vi "Facade.vi"(0 "Data In":T5, 2 "Display State In":T2={"WebView2 Ref"=refnum, "event callback refnum"=refnum, "Events"={"Navigation Complete Event"=refnum, "Source Changed Event"=refnum, "Document Title Changed Event"=refnum, "Status Bar Text Changed"=refnum, "Web Message Received"=refnum, "Window Close Requested"=refnum}, "Paths"={"Webview2 Native"=path "C:/Users/kleins/Desktop/webview2/microsoft.web.webview2.1.0.1370.28/build/native", "Edge Application"=path "", "User Data"=path ""}}, 3 "Container State":T4) -> (6 "Data Out":T5, 7 "Display State Out":T2={"WebView2 Ref"=refnum, "event callback refnum"=refnum, "Events"={"Navigation Complete Event"=refnum, "Source Changed Event"=refnum, "Document Title Changed Event"=refnum, "Status Bar Text Changed"=refnum, "Web Message Received"=refnum, "Window Close Requested"=refnum}, "Paths"={"Webview2 Native"=path "C:/Users/kleins/Desktop/webview2/microsoft.web.webview2.1.0.1370.28/build/native", "Edge Application"=path "", "User Data"=path ""}}, 8 "Action":T1)   [LabVIEW 2020, in "WebView2 Control.xctl"]
uses:
  WebView2 Control.xctl
  Data.ctl
  <vilib>/_xctls/Container State.ctl
  State.ctl
  C:/Users/kleins/Desktop/webview2/microsoft.web.webview2.1.0.1370.28/lib/net45/Microsoft.Web.WebView2.WinForms.dll
  microsoft.web.webview2.1.0.1370.28/lib/net45/Microsoft.Web.WebView2.WinForms.dll
  Paths.ctl
  <vilib>/_xctls/Action.ctl
  C:/Users/kleins/Desktop/webview2/microsoft.web.webview2.1.0.1370.28/lib/net45/Microsoft.Web.WebView2.Core.dll
  microsoft.web.webview2.1.0.1370.28/lib/net45/Microsoft.Web.WebView2.Core.dll
  <vilib>/_xctls/XControlSupport.lvlib
panel:
  in  "WebView2":refnum<k24>(container)
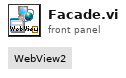
[diagram p1: front panel]
types:
  T1 = typedef "XControlSupport.lvlib/Action.ctl" = cluster{"Data Changed?":bool, "State Changed?":bool, "Action Name":string}
  T2 = typedef "WebView2 Control.xctl/State.ctl" = cluster{"WebView2 Ref":refnum<data-value>, "event callback refnum":refnum<k27>, "Events":cluster{"Navigation Complete Event":refnum<user-event>, "Source Changed Event":refnum<user-event>, "Document Title Changed Event":refnum<user-event>, "Status Bar Text Changed":refnum<user-event>, "Web Message Received":refnum<user-event>, "Window Close Requested":refnum<user-event>}, "Paths":T3}
  T3 = typedef "WebView2 Control.xctl/Paths.ctl" = cluster{"Webview2 Native":path, "Edge Application":path, "User Data":path}
  T4 = typedef "XControlSupport.lvlib/Container State.ctl" = cluster{"Indicator?":bool, "Run Mode?":bool, " Refnum":refnum<vi>}
  T5 = typedef "WebView2 Control.xctl/Data.ctl" = string
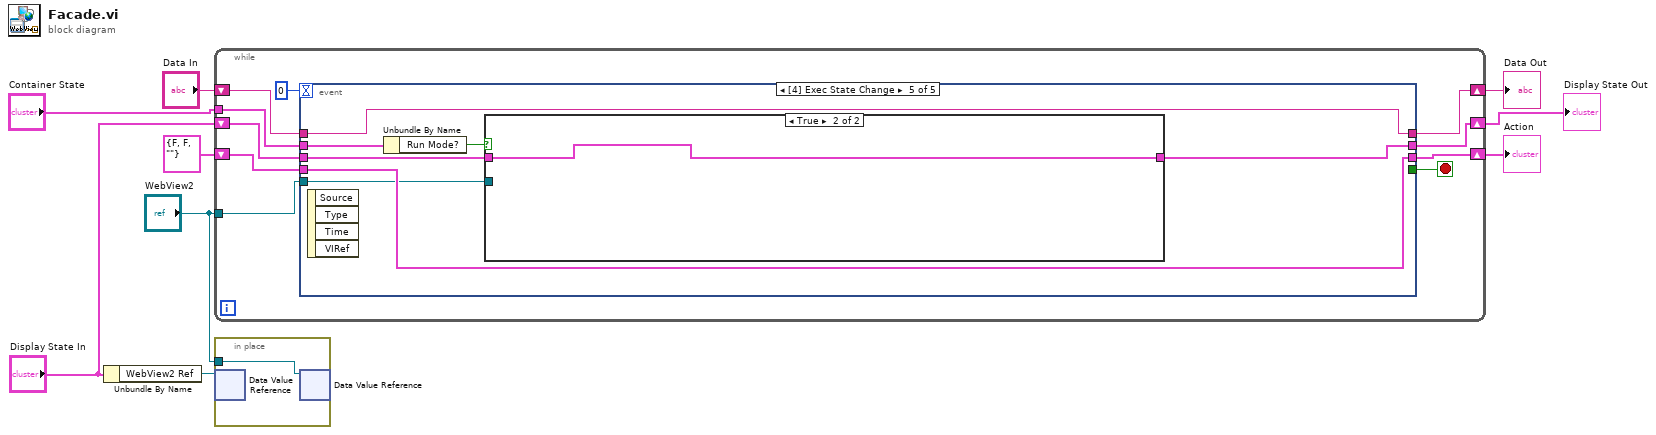
[diagram p0: block diagram]
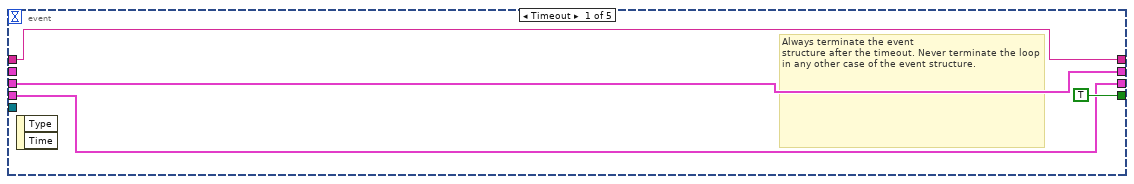
[diagram p2: hidden frame]
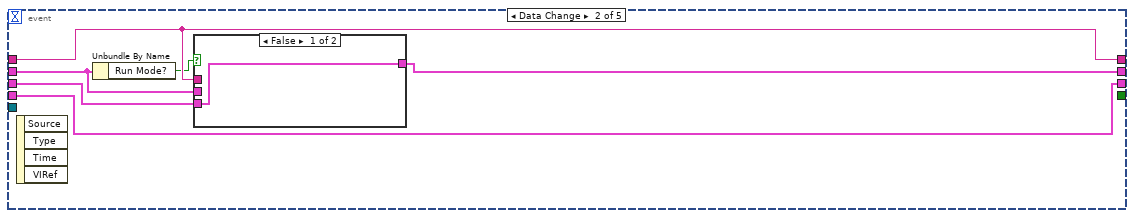
[diagram p3: hidden frame]
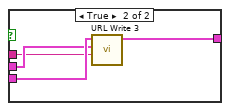
[diagram p4: hidden frame]
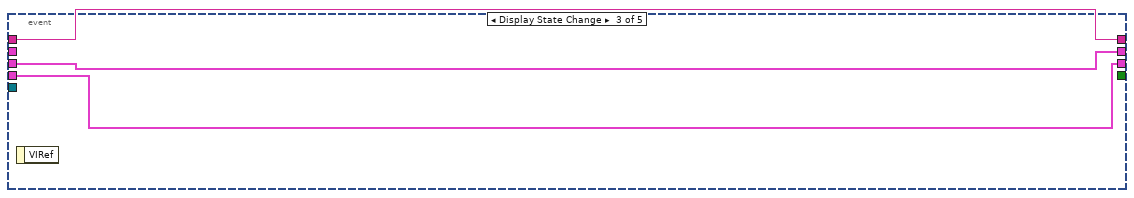
[diagram p5: hidden frame]
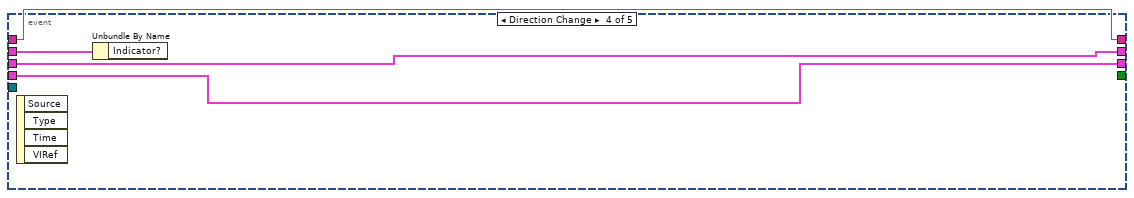
[diagram p6: hidden frame]
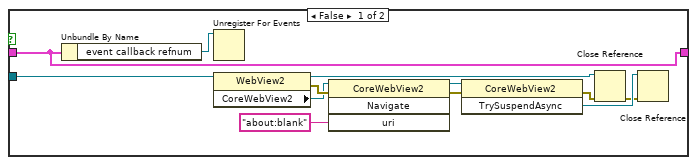
[diagram p7: hidden frame]
diagram:
  n1 = Unbundle By Name("Display State In") -> ("WebView2 Ref"=w2:refnum<data-value>)
  n2 = while {
    shift-right: [w18] -> w6
    shift-left: "Display State In" -> [w19]
    tunnel: "Container State" -> [w15]
    shift-right: [w13] -> w9
    shift-left: "Data In" -> [w14]
    shift-right: [w11] -> w5
    shift-left: T1 {"Data Changed?"=FALSE, "State Changed?"=FALSE, "Action Name"=""} ("Action") -> [w12]
    tunnel: "WebView2" -> [w10]
    stop <- w17 stop-if-true
    n3 = event shown="[4] Exec State Change" {
      selector: _ -> [_ _ _ _ _]
      dyn-events: _ -> [_ _ _ _ _]
      timeout: 0 -> [_ _ _ _ _]
      tunnel: w19 -> [w21 w27 w37 w40 w43]
      tunnel: [w21 w24 w37 w40 w42] -> w18
      tunnel: [TRUE _ _ _ _] -> w17
      tunnel: w15 -> [_ w25 _ w41 w48]
      tunnel: w14 -> [w20 w28 w36 w39 w47]
      tunnel: [w20 w28 w36 w39 w47] -> w13
      tunnel: [w22 w29 w35 w38 w46] -> w11
      tunnel: w12 -> [w22 w29 w35 w38 w46]
      tunnel: w10 -> [_ _ _ _ w45]
      event Timeout {
        # "Always terminate the event\nstructure after the timeout. Never terminate the loop in any other case of the event structure."
        n4 = event-data() -> ()  [unwired: 1 in, 2 out]
      }
      event Data Change {
        n5 = event-data() -> ()  [unwired: 1 in, 4 out]
        n6 = Unbundle By Name(w25) -> ("Run Mode?"=w26:bool)
        n7 = case shown="False" w26 {
          tunnel: w28 -> [_ w32]
          tunnel: w27 -> [w30 w34]
          tunnel: w25 -> [_ w33]
          tunnel: [w30 w31] -> w24
          frame False {
          }
          frame True {
            n8 = call "URL Write 3.vi"("Value"=w32, "Container State"=w33, "Display State In"=w34) -> ("Display State Out"=w31:T2)  [unwired: 3 in, 1 out]
          }
        }
      }
      event Display State Change {
        n9 = event-data() -> ()  [unwired: 1 in, 1 out]
      }
      event Direction Change {
        n10 = event-data() -> ()  [unwired: 1 in, 4 out]
        n11 = Unbundle By Name(w41) -> ()  [unwired: 1 out]
      }
      event Exec State Change {
        n12 = event-data() -> ()  [unwired: 1 in, 4 out]
        n13 = Unbundle By Name(w48) -> ("Run Mode?"=w44:bool)
        n14 = case shown="True" w44 {
          tunnel: w45 -> [w53 _]
          tunnel: w43 -> [w50 w61]
          tunnel: [w50 w61] -> w42
          frame False {
            n15 = Unbundle By Name(w50) -> ("event callback refnum"=w49:refnum<k27>)
            n16 = Unregister For Events(event registration refnum=w49) -> ()  [unwired: 1 in, 1 out]
            n17 = property class="WebView2"(reference=w53) -> (reference out=w52:refnum<k24>, error out=w59:errorcluster, "CoreWebView2"=w56:refnum<k24>)  [unwired: 1 in]
            n18 = invoke class="CoreWebView2" method="Navigate"(reference=w56, error in=w59, "uri"="about:blank") -> (reference out=w55:refnum<k24>, error out=w57:errorcluster)  [unwired: 1 in, 2 out]
            n19 = invoke class="CoreWebView2" method="TrySuspendAsync"(reference=w55, error in=w57) -> (error out=w51:errorcluster, "TrySuspendAsync"=w60:refnum<k24>)  [unwired: 1 in, 1 out]
            n20 = Close Reference(reference=w52, error in (no error)=w51) -> (error out=w58:errorcluster)
            n21 = Close Reference(reference=w60, error in (no error)=w58) -> ()  [unwired: 1 out]
          }
          frame True {
          }
        }
      }
    }
  }
  "Display State Out" <- w6
  "Data Out" <- w9
  "Action" <- w5
  n22 = in-place {
    in-place-border: "WebView2" -> [w62]
    n23 = in-place-dvr #1(w2) -> ()  [unwired: 2 out]
    n24 = in-place-dvr #1(w62) -> ()  [unwired: 2 out]
  }
